vi "DefaultIconGlyphData.vi"() -> (0 "defaultImageInfo":T2(array[cluster]))   [LabVIEW 2020]
doc: "Default glyphs installed in <Documents>\\LabVIEW Data\\Glyphs upon first launch."
uses:
  <vilib>/picture/picture.llb/imagedata.ctl
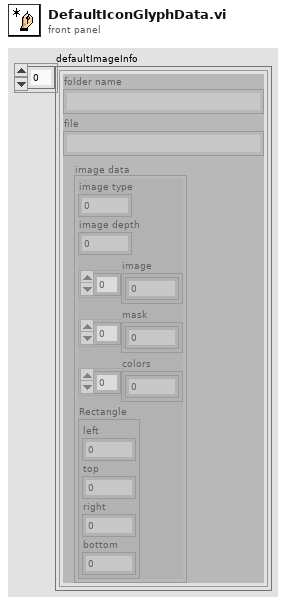
[diagram p1: front panel]
types:
  T1 = typedef "imagedata.ctl" = cluster{"image type":i32, "image depth":i32, "image":u8[], "mask":u8[], "colors":u32[], "Rectangle":cluster{"left":i16, "top":i16, "right":i16, "bottom":i16}}
  T2 = cluster{"folder name":string, "file":string, "image data":T1}[]
  T3 = cluster{"folder name":string, "file":string, "image data":T1}
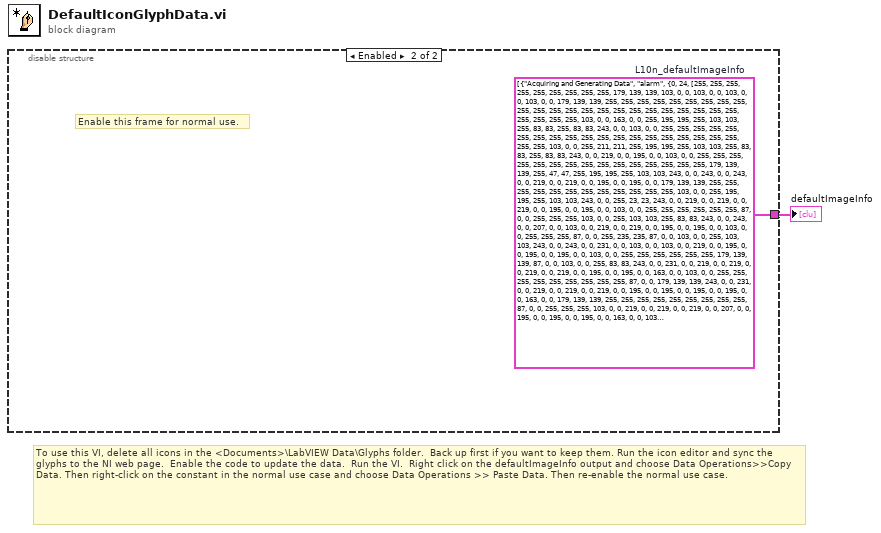
[diagram p0: block diagram]
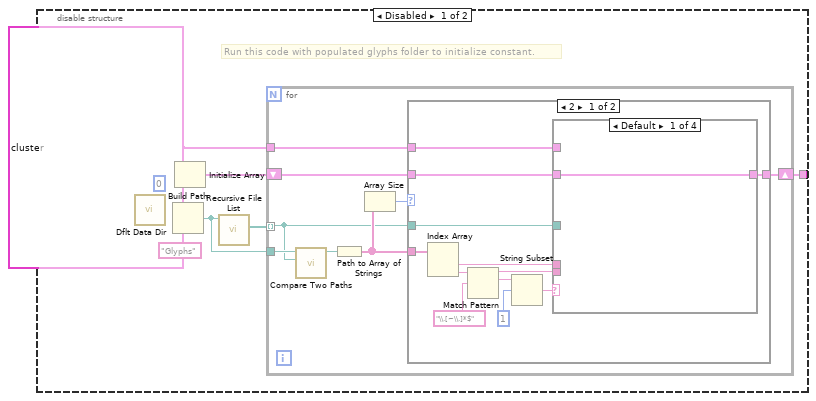
[diagram p2: hidden frame]
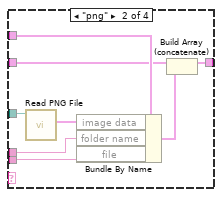
[diagram p3: hidden frame]
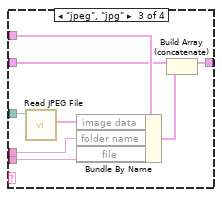
[diagram p4: hidden frame]
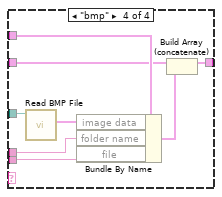
[diagram p5: hidden frame]
diagram:
  # "To use this VI, delete all icons in the <Documents>\\LabVIEW Data\\Glyphs folder.  Back up first if you want to keep them. Run the icon editor and sync the glyphs to the NI web page.  Enable the code to update the data.  Run the VI.  Right click on the defaultImageInfo output and choose Data Operations>>Copy Data. Then right-click on the constant in the normal use case and choose Data Operations >> Paste Data. Then re-enable the normal use case."
  n1 = disable-structure shown="Enabled" {
    disable-tunnel: [w2 w56] -> w1
    frame Disabled {
      w4 = T3 {"folder name"="Acquiring and Generating Data", "file"="ChnGroup", "image data"={"image type"=0, "image depth"=24, "image"=array[3072 elements], "mask"=[0, 0, 0, 0, 224, 0, 0, 0, 224, 0, 0, 0, 224, 0, 0, 0, 238, 0, 0, 0, 238, 0, 0, 0, 238, 0, 0, 0, 238, 224, 0, 0, 238, 224, 0, 0, 238, 224, 0, 0, 238, 238, 0, 0, 238, 238, 0, 0, 238, 238, 0, 0, 238, 238, 0, 0, 238, 238, 0, 0, 0, 0, 0, 0, 0, 0, 0, 0, 0, 0, 0, 0, 0, 0, 0, 0, 0, 0, 0, 0, 0, 0, 0, 0, 0, 0, 0, 0, 0, 0, 0, 0, 0, 0, 0, 0, 0, 0, 0, 0, 0, 0, 0, 0, 0, 0, 0, 0, 0, 0, 0, 0, 0, 0, 0, 0, 0, 0, 0, 0, 0, 0, 0, 0, 0, 0, 0, 0], "colors"=[], "Rectangle"={"left"=0, "top"=0, "right"=32, "bottom"=32}}} ("cluster")
      # "Run this code with populated glyphs folder to initialize constant."
      n2 = call <vilib>:"Dflt Data Dir.vi"() -> ("App:Default Data Directory"=w9:path)
      n3 = Build Path(base path=w9, name or relative path="Glyphs") -> (appended path=w6:path)
      n4 = Initialize Array(w4, 0 ("dimension size")) -> (w3:T2)
      n5 = call <vilib>:"Recursive File List.vi"("Folder Path"=w6) -> ("All Files in Dir"=w7:path[])  [unwired: 6 in, 4 out]
      n6 = for {
        tunnel: w7 -> [w10] mode=indexing
        tunnel: w6 -> [w17]
        tunnel: w4 -> [w15]
        shift-right: [w13] -> w2
        shift-left: w3 -> [w12]
        n7 = call <vilib>:"Compare Two Paths.vi"("Path 2"=w10, "Path 1"=w17) -> ("Relative Path from 1 to 2"=w16:path)  [unwired: 6 in, 3 out]
        n8 = Path to Array of Strings(0:w16) -> (2:w11:string[])  [unwired: 1 out]
        n9 = Array Size(array=w11) -> (size(s)=w14:i32)
        n10 = case shown="2" w14 {
          tunnel: w15 -> [w20 _]
          tunnel: [w18 w55] -> w13
          tunnel: w12 -> [w19 w55]
          tunnel: w11 -> [w29 _]
          tunnel: w10 -> [w21 _]
          frame 2 {
            n11 = Index Array(array=w29) -> (element #1=w22:string, element #2=w25:string)  [unwired: 2 in]
            n12 = Match Pattern(string=w25, regular expression="\\.[~\\.]*$") -> (before substring=w23:string, match substring=w28:string)  [unwired: 3 out]
            n13 = String Subset(string=w28, offset (0)=1) -> (substring=w24:string)  [unwired: 1 out]
            n14 = case shown="Default" w24 {
              tunnel: w23 -> [_ w35 w43 w51]
              tunnel: w22 -> [_ w34 w42 w50]
              tunnel: w21 -> [_ w38 w46 w54]
              tunnel: w20 -> [_ w37 w45 w53]
              tunnel: w19 -> [w30 w33 w41 w49]
              tunnel: [w30 w31 w39 w47] -> w18
              frame Default {
              }
              frame "png" {
                n15 = call <vilib>:"Read PNG File.vi"("path to PNG file"=w38) -> ("image data"=w36:T1)  [unwired: 8 in, 2 out]
                n16 = Bundle By Name(cluster=w37, "image data"=w36, "folder name"=w34, "file"=w35) -> (w32:T3)
                n17 = Build Array (concatenate)(w33, w32) -> (w31:T2)
              }
              frame "jpeg", "jpg" {
                n18 = call <vilib>:"Read JPEG File.vi"("path to JPEG file"=w46) -> ("image data"=w44:T1)  [unwired: 8 in, 2 out]
                n19 = Bundle By Name(cluster=w45, "image data"=w44, "folder name"=w42, "file"=w43) -> (w40:T3)
                n20 = Build Array (concatenate)(w41, w40) -> (w39:T2)
              }
              frame "bmp" {
                n21 = call <vilib>:"Read BMP File.vi"("path to BMP file"=w54) -> ("image data"=w52:T1)  [unwired: 8 in, 2 out]
                n22 = Bundle By Name(cluster=w53, "image data"=w52, "folder name"=w50, "file"=w51) -> (w48:T3)
                n23 = Build Array (concatenate)(w49, w48) -> (w47:T2)
              }
            }
          }
          frame Default {
          }
        }
      }
    }
    frame Enabled {
      w56 = T2 [{"folder name"="Acquiring and Generating Data", "file"="alarm", "image data"={"image type"=0, "image depth"=24, "image"=[255, 255, 255, 255, 255, 255, 255, 255, 255, 179, 139, 139, 103, 0, 0, 103, 0, 0, 103, 0, 0, 103, 0, 0, 179, 139, 139, 255, 255, 255, 255, 255, 255, 255, 255, 255, 255, 255, 255, 255, 255, 255, 255, 255, 255, 255, 255, 255, 255, 255, 255, 255, 255, 255, 103, 0, 0, 163, 0, 0, 255, 195, 195, 255, 103, 103, 255, 83, 83, 255, 83, 83, 243, 0, 0, 103, 0, 0, 255, 255, 255, 255, 255, 255, 255, 255, 255, 255, 255, 255, 255, 255, 255, 255, 255, 255, 255, 255, 255, 103, 0, 0, 255, 211, 211, 255, 195, 195, 255, 103, 103, 255, 83, 83, 255, 83, 83, 243, 0, 0, 219, 0, 0, 195, 0, 0, 103, 0, 0, 255, 255, 255, 255, 255, 255, 255, 255, 255, 255, 255, 255, 255, 255, 255, 179, 139, 139, 255, 47, 47, 255, 195, 195, 255, 103, 103, 243, 0, 0, 243, 0, 0, 243, 0, 0, 219, 0, 0, 219, 0, 0, 195, 0, 0, 195, 0, 0, 179, 139, 139, 255, 255, 255, 255, 255, 255, 255, 255, 255, 255, 255, 255, 103, 0, 0, 255, 195, 195, 255, 103, 103, 243, 0, 0, 255, 23, 23, 243, 0, 0, 219, 0, 0, 219, 0, 0, 219, 0, 0, 195, 0, 0, 195, 0, 0, 103, 0, 0, 255, 255, 255, 255, 255, 255, 87, 0, 0, 255, 255, 255, 103, 0, 0, 255, 103, 103, 255, 83, 83, 243, 0, 0, 243, 0, 0, 207, 0, 0, 103, 0, 0, 219, 0, 0, 219, 0, 0, 195, 0, 0, 195, 0, 0, 103, 0, 0, 255, 255, 255, 87, 0, 0, 255, 235, 235, 87, 0, 0, 103, 0, 0, 255, 103, 103, 243, 0, 0, 243, 0, 0, 231, 0, 0, 103, 0, 0, 103, 0, 0, 219, 0, 0, 195, 0, 0, 195, 0, 0, 195, 0, 0, 103, 0, 0, 255, 255, 255, 255, 255, 255, 179, 139, 139, 87, 0, 0, 103, 0, 0, 255, 83, 83, 243, 0, 0, 231, 0, 0, 219, 0, 0, 219, 0, 0, 219, 0, 0, 219, 0, 0, 195, 0, 0, 195, 0, 0, 163, 0, 0, 103, 0, 0, 255, 255, 255, 255, 255, 255, 255, 255, 255, 87, 0, 0, 179, 139, 139, 243, 0, 0, 231, 0, 0, 219, 0, 0, 219, 0, 0, 219, 0, 0, 195, 0, 0, 195, 0, 0, 195, 0, 0, 195, 0, 0, 163, 0, 0, 179, 139, 139, 255, 255, 255, 255, 255, 255, 255, 255, 255, 87, 0, 0, 255, 255, 255, 103, 0, 0, 219, 0, 0, 219, 0, 0, 219, 0, 0, 207, 0, 0, 195, 0, 0, 195, 0, 0, 195, 0, 0, 163, 0, 0, 103, 0, 0, 255, 255, 255, 255, 255, 255, 255, 255, 255, 87, 0, 0, 179, 139, 139, 255, 255, 255, 255, 255, 255, 103, 0, 0, 219, 0, 0, 207, 0, 0, 195, 0, 0, 195, 0, 0, 195, 0, 0, 195, 0, 0, 103, 0, 0, 255, 255, 255, 255, 255, 255, 255, 255, 255, 87, 0, 0, 87, 0, 0, 255, 255, 255, 255, 255, 255, 255, 255, 255, 255, 255, 255, 179, 139, 139, 103, 0, 0, 103, 0, 0, 103, 0, 0, 103, 0, 0, 179, 139, 139, 255, 255, 255, 255, 255, 255, 255, 255, 255, 87, 0, 0, 87, 0, 0, 255, 255, 255, 255, 255, 255, 255, 255, 255, 255, 255, 255, 255, 255, 255, 255, 255, 255, 255, 255, 255, 87, 0, 0, 220, 220, 220, 87, 0, 0, 255, 255, 255, 255, 255, 255, 255, 255, 255, 87, 0, 0, 87, 0, 0, 255, 255, 255, 255, 255, 255, 255, 255, 255, 255, 255, 255, 255, 255, 255, 255, 255, 255, 255, 255, 255, 51, 0, 47, 47, 83, 47, 87, 0, 0, 87, 0, 0, 87, 0, 0, 87, 0, 0, 87, 0, 0, 87, 0, 0, 255, 255, 255, 255, 255, 255, 255, 255, 255, 255, 255, 255, 255, 255, 255, 255, 255, 255, 255, 255, 255, 255, 255, 255, 0, 0, 0, 128, 128, 128, 128, 128, 128, 128, 128, 128, 128, 128, 128, 128, 128, 128, 179, 139, 139, 87, 0, 0, 255, 255, 255, 255, 255, 255, 255, 255, 255, 255, 255, 255, 255, 255, 255, 255, 255, 255, 255, 255, 255, 255, 255, 255, 255, 255, 255, 0, 0, 0, 87, 0, 0, 87, 0, 0, 87, 0, 0, 87, 0, 0, 87, 0, 0, 255, 255, 255, 255, 255, 255, 255, 255, 255, 255, 255, 255, 255, 255, 255], "mask"=[], "colors"=[], "Rectangle"={"left"=0, "top"=0, "right"=16, "bottom"=16}}}, ...(934 in all)]  # L10n_defaultImageInfo
      # "Enable this frame for normal use."
    }
  }
  "defaultImageInfo" <- w1
